vi "Get Used Encoding.vi"(8 "error in (no error)":errorcluster, 11 "CConfig Encoding in":refnum<class "CConfig Encoding.lvclass">) -> (0 "error out":errorcluster, 3 "CConfig Encoding out":refnum<class "CConfig Encoding.lvclass">)   [LabVIEW 2013, in "CConfig Encoding.lvclass"]
doc: "Copyright 2018, Carya Automatisering, Wiebe Walstra."
uses:
  CConfig Encoding.lvclass
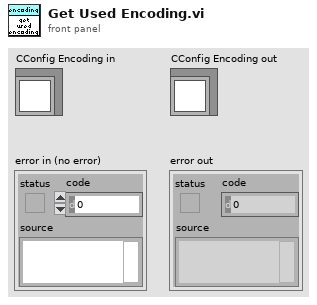
[diagram p1: front panel]
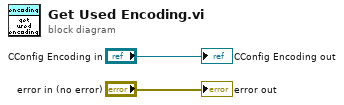
[diagram p0: block diagram]
diagram:
  "error out" <- "error in (no error)"
  "CConfig Encoding out" <- "CConfig Encoding in"
